vi "2019-05-013_Lecture5_Challenges.vi"() -> ()   [LabVIEW 2018]
panel:
  in  "정지 3":bool
  out "y":i8(slide) scale=1.0..100.0
  out "y":i8(slide) scale=1.0..100.0
  in  "정지 2":bool
  in  "초기화":bool
  in  "증가":bool
  out "탱크":dbl(slide) scale=0.0..10.0
  out "z":dbl
  in  "y":dbl
  in  "x":dbl
  in  "/":bool
  in  "*":bool
  in  "-":bool
  in  "+":bool
  in  "정지":bool
  in  "도전과제":enum16{"1", "2", "3", "4"}(ring)
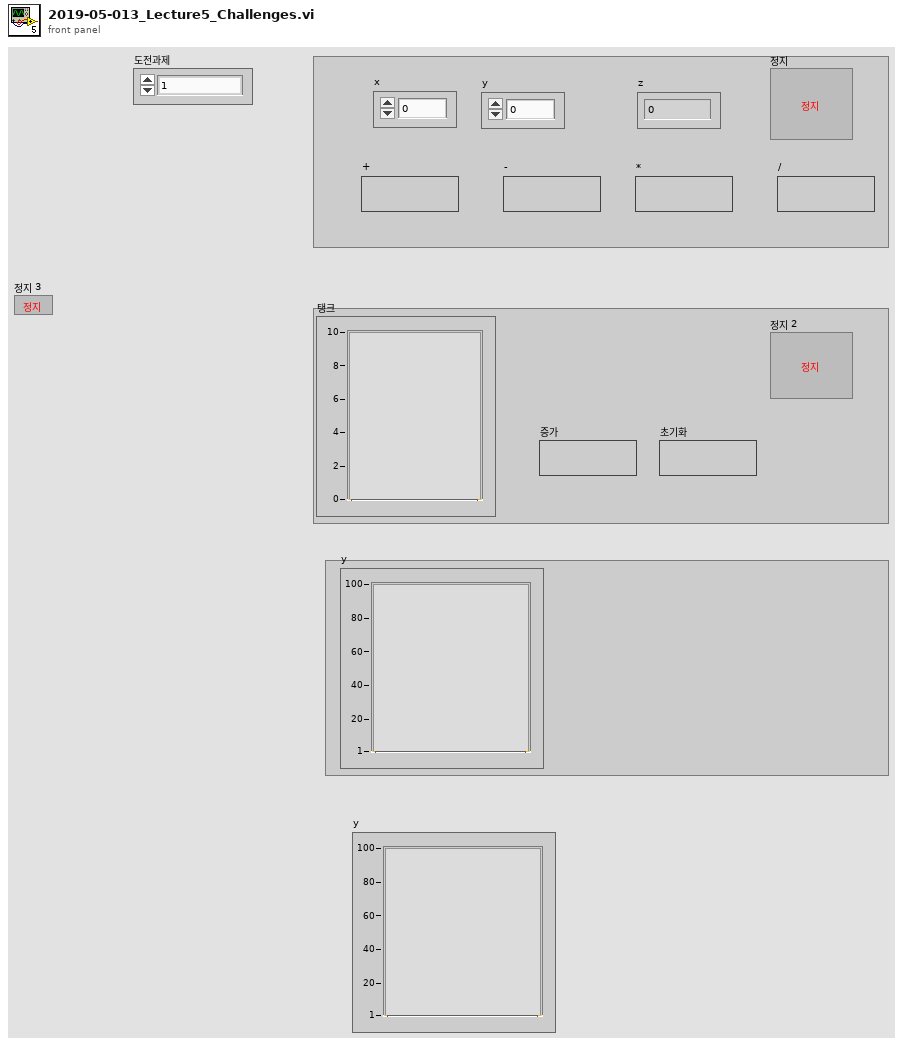
[diagram p1: front panel]
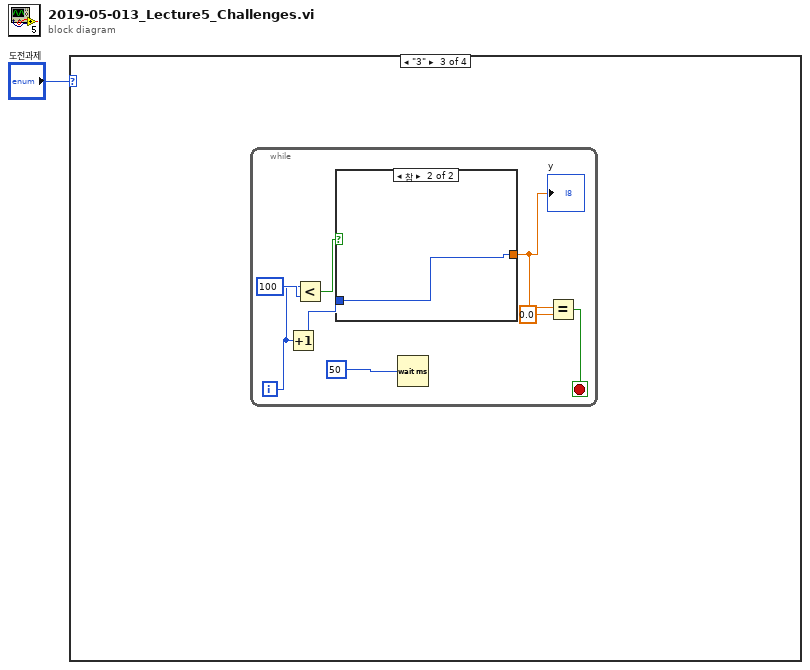
[diagram p0: block diagram]
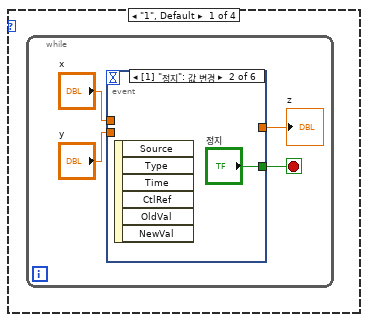
[diagram p2: hidden frame]
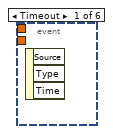
[diagram p3: hidden frame]
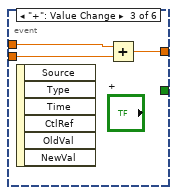
[diagram p4: hidden frame]
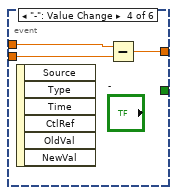
[diagram p5: hidden frame]
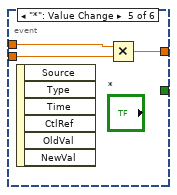
[diagram p6: hidden frame]
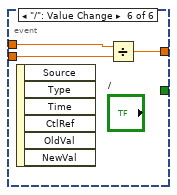
[diagram p7: hidden frame]
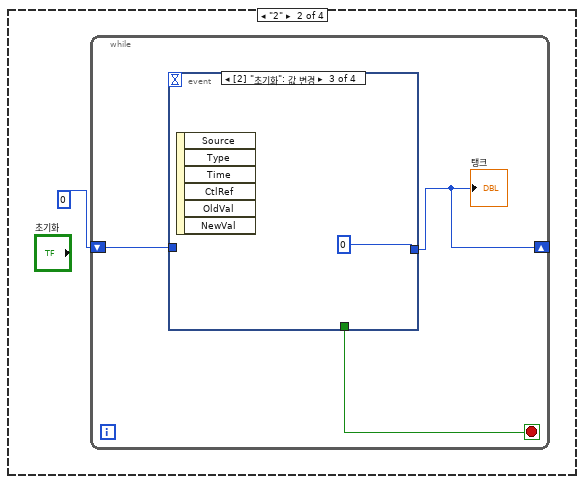
[diagram p8: hidden frame]
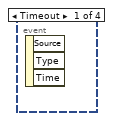
[diagram p9: hidden frame]
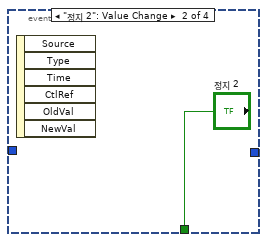
[diagram p10: hidden frame]
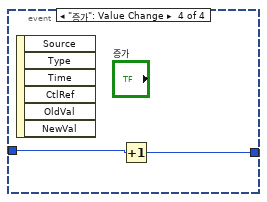
[diagram p11: hidden frame]
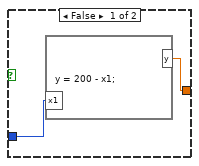
[diagram p12: hidden frame]
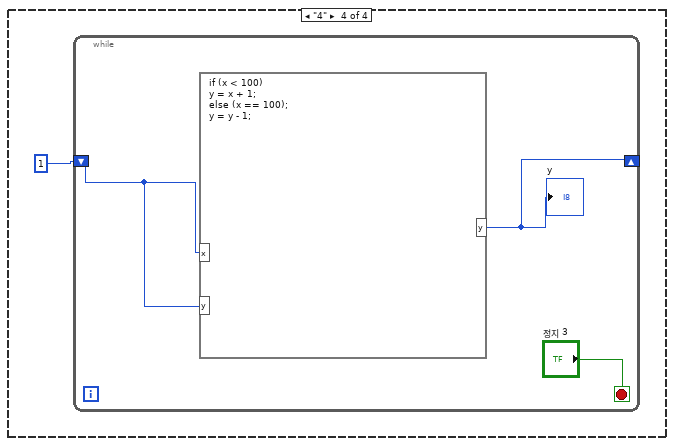
[diagram p13: hidden frame]
diagram:
  n1 = case shown="\"3\"" "도전과제" {
    frame "1", Default {
      n2 = while {
        stop <- w5 stop-if-true
        n3 = event shown="[1] \"정지\": 값 변경" {
          selector: _ -> [_ _ _ _ _ _]
          dyn-events: _ -> [_ _ _ _ _ _]
          timeout: _ -> [_ _ _ _ _ _]
          tunnel: [_ "정지" _ _ _ _] -> w5
          tunnel: "x" -> [_ _ w9 w12 w15 w18]
          tunnel: "y" -> [_ _ w8 w11 w14 w17]
          tunnel: [_ _ w7 w10 w13 w16] -> w2
          event Timeout {
            n4 = event-data() -> ()  [unwired: 1 in, 3 out]
          }
          event "정지": Value Change {
            n5 = event-data() -> ()  [unwired: 1 in, 6 out]
          }
          event "+": Value Change {
            n6 = event-data() -> ()  [unwired: 1 in, 6 out]
            n7 = Add(x=w9, y=w8) -> (x+y=w7:dbl)
          }
          event "-": Value Change {
            n8 = event-data() -> ()  [unwired: 1 in, 6 out]
            n9 = Subtract(x=w12, y=w11) -> (x-y=w10:dbl)
          }
          event "*": Value Change {
            n10 = event-data() -> ()  [unwired: 1 in, 6 out]
            n11 = Multiply(x=w15, y=w14) -> (x*y=w13:dbl)
          }
          event "/": Value Change {
            n12 = event-data() -> ()  [unwired: 1 in, 6 out]
            n13 = Divide(x=w18, y=w17) -> (x/y=w16:dbl)
          }
        }
        "z" <- w2
      }
    }
    frame "2" {
      n14 = while {
        shift-right: [w20] -> _
        shift-left: 0 -> [w21]
        stop <- w22 stop-if-true
        n15 = event shown="[2] \"초기화\": 값 변경" {
          selector: _ -> [_ _ _ _]
          dyn-events: _ -> [_ _ _ _]
          timeout: _ -> [_ _ _ _]
          tunnel: [_ "정지 2" _ _] -> w22
          tunnel: w21 -> [_ _ _ w26]
          tunnel: [_ _ 0 w25] -> w20
          event Timeout {
            n16 = event-data() -> ()  [unwired: 1 in, 3 out]
          }
          event "정지 2": Value Change {
            n17 = event-data() -> ()  [unwired: 1 in, 6 out]
          }
          event "초기화": Value Change {
            n18 = event-data() -> ()  [unwired: 1 in, 6 out]
          }
          event "증가": Value Change {
            n19 = event-data() -> ()  [unwired: 1 in, 6 out]
            n20 = Increment(x=w26) -> (x+1=w25:i32)
          }
        }
        "탱크" <- w20
      }
    }
    frame "3" {
      n21 = while {
        i -> [w27]
        stop <- w28 stop-if-true
        n22 = Increment(x=w27) -> (x+1=w31:i32)
        n23 = Less?(x=w27, y=100 ("x")) -> (x < y?=w33:bool)
        n24 = case shown="참" w33 {
          tunnel: [w35 w37] -> w30
          tunnel: w31 -> [w36 w37]
          frame False {
            n25 = formula code="y = 200 - x1;"("x1"=w36) -> ("y"=w35:dbl)
          }
          frame True {
          }
        }
        "y" <- w30
        n26 = Wait (ms)(milliseconds to wait=u32 50 ("대기 시간 (ms)")) -> ()  [unwired: 1 out]
        n27 = Equal?(x=w30, y=0.0) -> (x = y?=w28:bool)
      }
    }
    frame "4" {
      n28 = while {
        shift-right: [w40] -> _
        shift-left: 1 -> [w41]
        stop <- "정지 3" stop-if-true
        n29 = formula code="if (x < 100)\ny = x + 1;\nelse (x == 100);\ny = y - 1;"("x"=w41, "y"=w41) -> ("y"=w40:i32)
        "y" <- w40
      }
    }
  }
